vi "LINX - PmodGYRO.vi"() -> ()   [LabVIEW 2020]
doc: "PmodGYRO\n\nThis example demonstrates how to read the angular velocity values from the PmodGYRO.\n\nInstructions:\n1. Select the COM Port associated with the LINX device\n2. Select the I2C Channel that the Pmod is connected to.\n3. Select the Slave Address for the Pmod (default 0x69)\n4. Select the desired resolution.\n5. Click the Run Arrow."
uses:
  vi.lib/MakerHub/LINX/LMH-LINX.lvlib
  vi.lib/MakerHub/LINX/Public/Sensors/Pmods/GYRO/PmodGYRO.lvlib
panel:
  out "Waveform Chart":cluster{"X":i16, "Y":i16, "Z":i16}(graph)
  in  "Stop Button":bool
  out "Gyro XYZ (degrees/sec)":cluster{"X":i16, "Y":i16, "Z":i16}
  in  "Resolution (dps)":enum16{"2000", "500", "250"}(ring)
  in  "Address":enum8{"0x68", "0x69"}(ring)=enum."0x69"
  in  "I2C Channel (0)":u8
  in  "Serial Port":refnum<visa-resource-name>="N/A"
  # "PmodGYRO\n\nThis example demonstrates how to read the angular velocity values from the PmodGYRO.\n\nInstructions:\n1. Select the COM Port associated with the LINX device\n2. Select the I2C Channel that the Pmod is connected to.\n3. Select the Slave Address for the Pmod (default 0x69)\n4. Select the desired resolution.\n5. Click the Run Arrow."
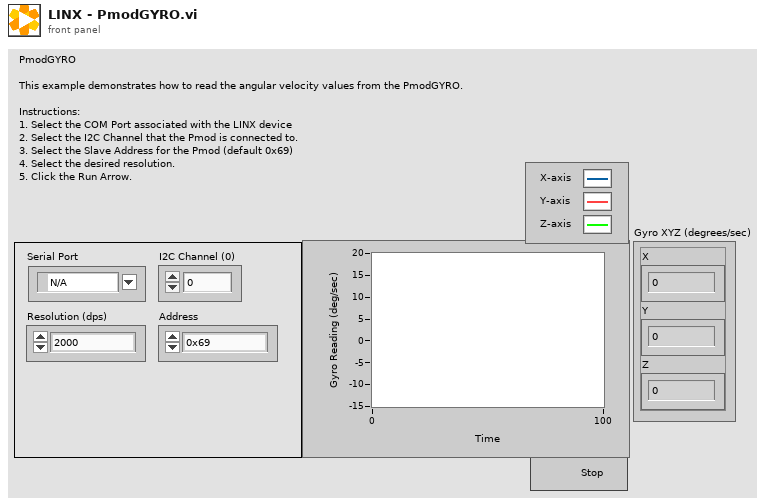
[diagram p1: front panel]
types:
  T1 = typedef "LMH-LINX.lvlib/LINX Ref.ctl" = cluster{"IO":T2, "Interface":T3, "LINX Device Config":T4}
  T2 = typedef "LMH-LINX.lvlib/Platform.ctl" = enum16{"Remote", "Local"}
  T3 = typedef "LMH-LINX.lvlib/Interface.ctl" = enum16{"Serial", "TCP"}
  T4 = typedef "Device.lvlib/LINX Device Config.ctl" = cluster{"Interface":T3, "COM Port":refnum<visa-resource-name>, "TCP Configuration":T5, "Device Family":u8, "Device ID":u8, "Device Name":string, "TCP Ref":refnum<k5>, "Channels":T6}
  T5 = typedef "Device.lvlib/TCP Config.ctl" = cluster{"IP Address":string, "Port":u16}
  T6 = typedef "LMH-LINX.lvlib/Channels.ctl" = cluster{"DI":u8[], "DO":u8[], "AI":u8[], "AO":u8[], "PWM":u8[], "QE":u8[], "UART":u8[], "I2C 2":u8[], "SPI":u8[], "CAN":u8[], "Servo":u8[], "AI Ref (V)":dbl, "AI Resolution (Bits)":u8, "AO Ref (V)":dbl, "AO Resolution (Bits)":u8}
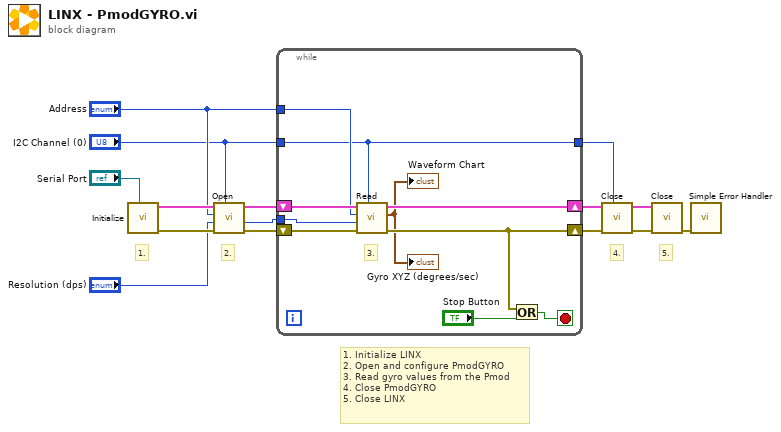
[diagram p0: block diagram]
diagram:
  # "1. Initialize LINX\n2. Open and configure PmodGYRO\n3. Read gyro values from the Pmod\n4. Close PmodGYRO\n5. Close LINX"
  # "5."
  # "4."
  # "2."
  # "1."
  n1 = call "Initialize.vi"("Serial Port"="Serial Port") -> ("Error Out"=w10:errorcluster, "LINX Resource"=w11:T1)  [unwired: 8 in, 1 out]
  n2 = call "Open.vi"("I2C Channel (0)"="I2C Channel (0)", "Error In"=w10, "Resolution (dps)"="Resolution (dps)", "I2C Slave Address (0x69)"="Address", "LINX Resource"=w11) -> ("Error Out"=w7:errorcluster, "Resolution (dps)"=w4:enum16{"2000", "500", "250"}, "LINX Resource"=w9:T1)  [unwired: 4 in]
  n3 = while {
    shift-right: [w24] -> w8
    shift-left: w9 -> [w25]
    shift-right: [w19] -> w6
    shift-left: w7 -> [w23]
    tunnel: w4 -> [w22]
    tunnel: "Address" -> [w21]
    tunnel: "I2C Channel (0)" -> [w20]
    tunnel: [w20] -> w1
    stop <- w17 stop-if-true
    # "3."
    n4 = call "Read.vi"("I2C Channel (0)"=w20, "Error In"=w23, "Resolution (dps)"=w22, "I2C Slave Address"=w21, "LINX Resource"=w25) -> ("Error Out"=w19:errorcluster, "Rotation(dps)"=→"Gyro XYZ (degrees/sec)" →"Waveform Chart":cluster{"X":i16, "Y":i16, "Z":i16}, "LINX Resource"=w24:T1)  [unwired: 4 in]
    n5 = Or(x=w19, y="Stop Button") -> (x .or. y?=w17:bool)
  }
  n6 = call "Close.vi"("I2C Channel (0)"=w1, "Error In"=w6, "LINX Resource"=w8) -> ("Error Out"=w13:errorcluster, "LINX Resource"=w12:T1)  [unwired: 7 in]
  n7 = call "Close.vi"("Error In"=w13, "LINX Resource"=w12) -> ("Error Out"=w15:errorcluster)  [unwired: 9 in]
  n8 = call <vilib>:"Simple Error Handler.vi"("error in (no error)"=w15) -> ()  [unwired: 4 in, 5 out]
